vi "Initalise.vi"(8 "error in (no error)":errorcluster, 11 "FPGA Interface":refnum<k20>) -> (0 "Encoder Index Position":i16, 2 "Error out":errorcluster, 3 "FPGA VI Reference Out":refnum<k20>, 4 "TDMS refnum out":refnum<k34>, 6 "Error log refnum out":refnum<file>)   [LabVIEW 2016]
uses:
  <vilib>/FPGAPlugInAG/Dynamic/niLvFpga_Reset_Dynamic.vi
  <vilib>/Utility/error.llb/Error Cluster From Error Code.vi
  <vilib>/rvi/errors/niLvFpgaAdjustHostInterfaceError.vi
  <vilib>/myRIO/Common/Instrument Driver Framework/Utilities/vis/FPGA Ref Manager.vi
  <vilib>/myRIO/Common/Instrument Driver Framework/Utilities/vis/Ref Counter.vi
  <vilib>/FPGAPlugInAG/Dynamic/niLvFpga_Run_Dynamic.vi
  <vilib>/rvi/interface/nirviMethod/nirviMethod.xnode
  <vilib>/rvi/interface/nirviReadWriteControl/nirviReadWriteControl.xnode
  <vilib>/rvi/interface/Simulation/niFpgaSimulationCallBeginRW.vi
  NiFpgaLv.dll
  <vilib>/myRIO/Instrument Drivers/Utilities/Utilities.lvlib
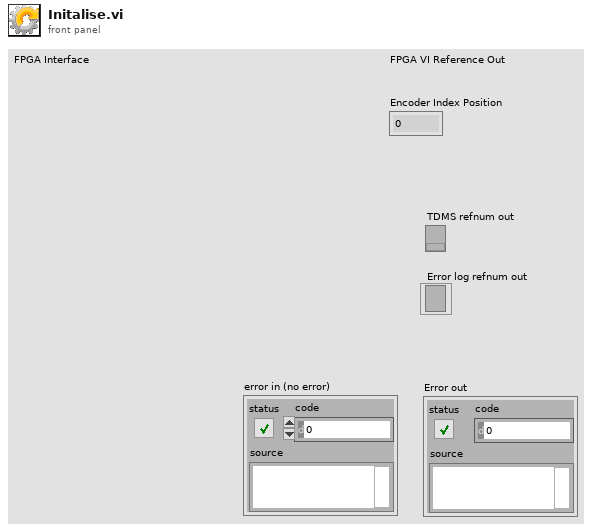
[diagram p1: front panel]
types:
  T1 = cluster{"Yaw":sgl, "Pitch":sgl, "Roll":sgl, "Lat":dbl, "Long":dbl, "Alt":dbl}
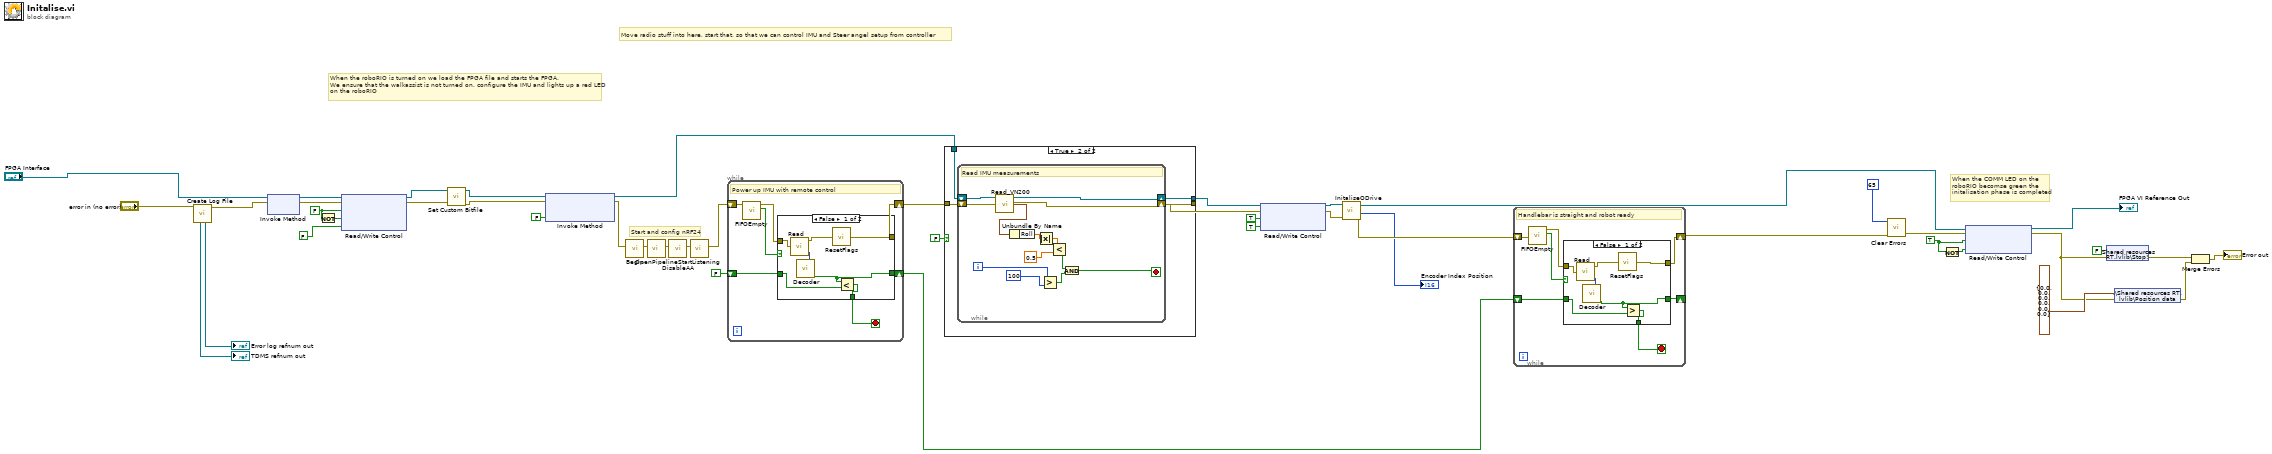
[diagram p0: block diagram]
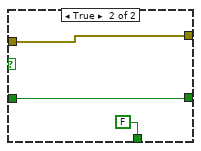
[diagram p3: hidden frame]
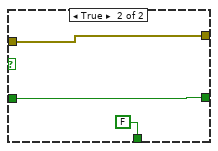
[diagram p4: hidden frame]
diagram:
  w35 = TRUE ("Steering motor on?")
  w32 = FALSE ("Steering motor on?")
  # "Start and config nRF24"
  # "Move radio stuff into here, start that, so that we can control IMU and Steer angel setup from controller"
  # "When the COMM LED on the\nroboRIO becomse green the\ninitalisation phase is completed"
  # "When the roboRIO is turned on we load the FPGA file and starts the FPGA.\nWe ensure that the walkassist is not turned on, configure the IMU and lights up a red LED\non the roboRIO"
  n1 = call "Create Log File.vi"("error in (no error)"="error in (no error)") -> ("error out"=w45:errorcluster, "Error log refnum out"=→"Error log refnum out":refnum<file>, "TDMS refnum out"=→"TDMS refnum out":refnum<k34>)  [unwired: 8 in]
  n2 = xnode "Invoke Method"("FPGA VI Reference In"="FPGA Interface", "error in"=w45) -> ("FPGA VI Reference Out"=w42:refnum<k20>, "error out"=w41:errorcluster)
  n3 = Not(x=w32) -> (.not. x?=w33:bool)
  n4 = xnode "Read/Write Control"("FPGA VI Reference In"=w42, "error in"=w41, "Comm LED Green"=w32, "Comm LED Red"=w33, "MotorsON"=FALSE ("Rear wheel motor OFF?")) -> ("FPGA VI Reference Out"=w13:refnum<k20>, "error out"=w14:errorcluster)
  n5 = call <vilib>:"Set Custom Bitfile.vi"("error in (no error)"=w14, "Custom FPGA Reference In"=w13) -> ("error out"=w12:errorcluster, "Custom FPGA Reference Out"=w11:refnum<k20>)  [unwired: 8 in]
  n6 = xnode "Invoke Method"("FPGA VI Reference In"=w11, "error in"=w12, "Wait Until Done (F)"=FALSE) -> ("FPGA VI Reference Out"=w20:refnum<k20>, "error out"=w22:errorcluster)
  n7 = call "Begin.vi"("error in (no error)"=w22) -> ("error out"=w25:errorcluster)  [unwired: 10 in]
  n8 = call "OpenPipeline.vi"("error in (no error)"=w25) -> ("error out"=w24:errorcluster)  [unwired: 10 in]
  n9 = call "DisableAA.vi"("error in (no error)"=w24) -> ("error out"=w23:errorcluster)  [unwired: 10 in]
  n10 = call "StartListening.vi"("error in (no error)"=w23) -> ("error out"=w21:errorcluster)  [unwired: 10 in]
  n11 = while {
    shift-right: [w50] -> w40
    shift-left: w21 -> [w52]
    shift-right: [w48] -> w17
    shift-left: FALSE -> [w49]
    stop <- w47 stop-if-true
    # "Power up IMU with remote control"
    n12 = call "FIFOEmpty.vi"("error in (no error)"=w52) -> ("RX_EMPTY"=w53:bool, "error out"=w51:errorcluster)  [unwired: 9 in]
    n13 = case shown="False" w53 {
      tunnel: w51 -> [w58 w63]
      tunnel: [w57 w63] -> w50
      tunnel: [w54 w62] -> w48
      tunnel: w49 -> [w55 w62]
      tunnel: [w56 FALSE] -> w47
      frame False {
        n14 = call "Read.vi"("error in (no error)"=w58) -> ("error out"=w59:errorcluster, "Data frame"=w60:u16[])  [unwired: 1 out]
        n15 = call "Decoder.vi"("Data frame"=w60) -> ("Kill Switch"=w54:bool)  [unwired: 17 in, 1 out]
        n16 = call "ResetFlags.vi"("error in (no error)"=w59) -> ("error out"=w57:errorcluster)
        n17 = Less?(x=w54, y=w55) -> (x < y?=w56:bool)
      }
      frame True {
      }
    }
  }
  n18 = case shown="True" FALSE {
    tunnel: w40 -> [w64 w69]
    tunnel: w20 -> [w65 w68]
    tunnel: [w65 w67] -> w10
    tunnel: [w64 w66] -> w9
    frame False {
    }
    frame True {
      n19 = while {
        shift-right: [w79] -> w67
        shift-left: w68 -> [w80]
        shift-right: [w77] -> w66
        shift-left: w69 -> [w78]
        i -> [w81]
        stop <- w82 stop-if-true
        # "Read IMU measurements"
        n20 = call "Read_VN200.vi"("FPGA Interface"=w80, "error in"=w78) -> ("FPGA Interface Out"=w79:refnum<k20>, "error out"=w77:errorcluster, "Position Data"=w74:T1)  [unwired: 11 in]
        n21 = Unbundle By Name(w74) -> ("Roll"=w73:sgl)
        n22 = Absolute Value(x=w73) -> (abs(x)=w72:sgl)
        n23 = Greater?(x=w81, y=100 ("x")) -> (0:w76:bool)
        n24 = Less?(x=w72, y=sgl 0.5) -> (x < y?=w70:bool)
        n25 = And(x=w70, y=w76) -> (x .and. y?=w82:bool)
      }
    }
  }
  n26 = xnode "Read/Write Control"("FPGA VI Reference In"=w10, "error in"=w9, "Comm LED Green"=TRUE, "Comm LED Red"=TRUE) -> ("FPGA VI Reference Out"=w8:refnum<k20>, "error out"=w7:errorcluster)
  n27 = call "InitaliseODrive.vi"("error in (no error)"=w7, "FPGA Interface in"=w8) -> ("error out"=w18:errorcluster, "Encoder Index Position"=→"Encoder Index Position":i16, "FPGA Interface out"=w3:refnum<k20>)  [unwired: 7 in]
  n28 = while {
    shift-right: [w86] -> w4
    shift-left: w18 -> [w88]
    shift-right: [w84] -> _
    shift-left: w17 -> [w85]
    stop <- w83 stop-if-true
    # "Handlebar is straight and robot ready"
    n29 = call "FIFOEmpty.vi"("error in (no error)"=w88) -> ("RX_EMPTY"=w89:bool, "error out"=w87:errorcluster)  [unwired: 9 in]
    n30 = case shown="False" w89 {
      tunnel: w87 -> [w94 w99]
      tunnel: [w93 w99] -> w86
      tunnel: [w90 w98] -> w84
      tunnel: w85 -> [w91 w98]
      tunnel: [w92 FALSE] -> w83
      frame False {
        n31 = call "Read.vi"("error in (no error)"=w94) -> ("error out"=w95:errorcluster, "Data frame"=w96:u16[])  [unwired: 1 out]
        n32 = call "Decoder.vi"("Data frame"=w96) -> ("Kill Switch"=w90:bool)  [unwired: 17 in, 1 out]
        n33 = call "ResetFlags.vi"("error in (no error)"=w95) -> ("error out"=w93:errorcluster)
        n34 = Greater?(x=w90, y=w91) -> (0:w92:bool)
      }
      frame True {
      }
    }
  }
  n35 = call <vilib>:"Clear Errors.vi"("error in (no error)"=w4, "specific error code to clear (0: all)"=65) -> ("error out"=w39:errorcluster)  [unwired: 4 in, 1 out]
  n36 = Not(x=w35) -> (.not. x?=w36:bool)
  n37 = xnode "Read/Write Control"("FPGA VI Reference In"=w3, "error in"=w39, "Comm LED Green"=w35, "Comm LED Red"=w36) -> ("FPGA VI Reference Out"=→"FPGA VI Reference Out":refnum<k20>, "error out"=w29:errorcluster)
  n38 = shared-variable ".\\Shared resources RT.lvlib\\Stop!"(FALSE ("Stop!"), error in=w29) -> (error out=w27:errorcluster)
  n39 = shared-variable ".\\Shared resources RT.lvlib\\Position data"(T1 {"Yaw"=0.0, "Pitch"=0.0, "Roll"=0.0, "Lat"=0.0, "Long"=0.0, "Alt"=0.0} ("Position data"), error in=w29) -> (error out=w26:errorcluster)
  n40 = Merge Errors(w27, w26) -> (→"Error out":errorcluster)
